vi "15-FindShortestPaths.vi"(5 "Risk Relief":refnum<vi>, 6 "Initial Position in":cluster{"Row":i32, "Col":i32}, 7 "Min Risk Relief":refnum<vi>, 8 "Min Risk Array in":i32[][](array[numeric]), 9 "Visited Array in":bool[][](array[boolean]), 10 "map in":T1(c390), 11 "Risk Array in":u8[][](array[numeric])) -> (0 "Min Risk Array out":i32[][](array[numeric]), 1 "Visited Array out":bool[][](array[boolean]), 2 "map out":T1(c390), 3 "Risk Array out":u8[][](array[numeric]))   [LabVIEW 2019, in "15.lvlib"]
uses:
  15.lvlib
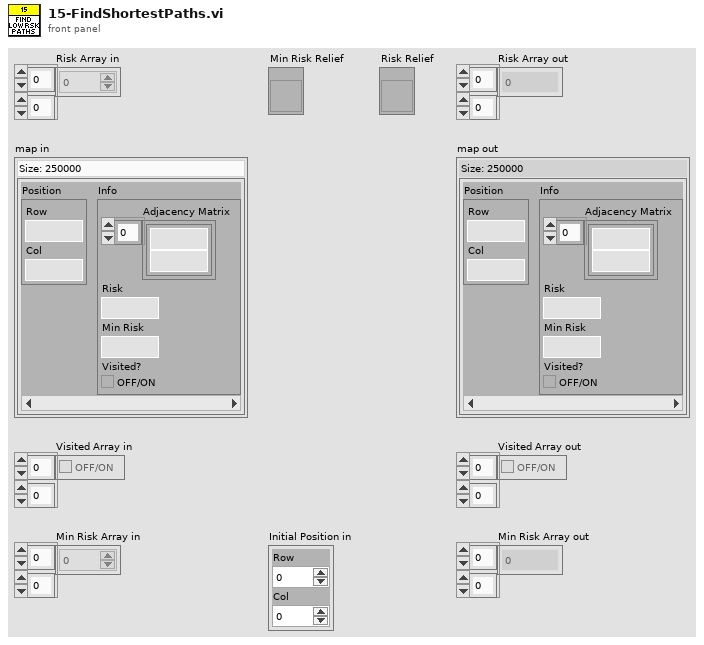
[diagram p1: front panel]
types:
  T1 = map{cluster{"Row":i32, "Col":i32}, cluster{"Adjacency Matrix":cluster{i32, i32}[], "Risk":u8, "Min Risk":i32, "Visited?":bool}}
  T2 = cluster{"Adjacency Matrix":cluster{i32, i32}[], "Risk":u8, "Min Risk":i32, "Visited?":bool}
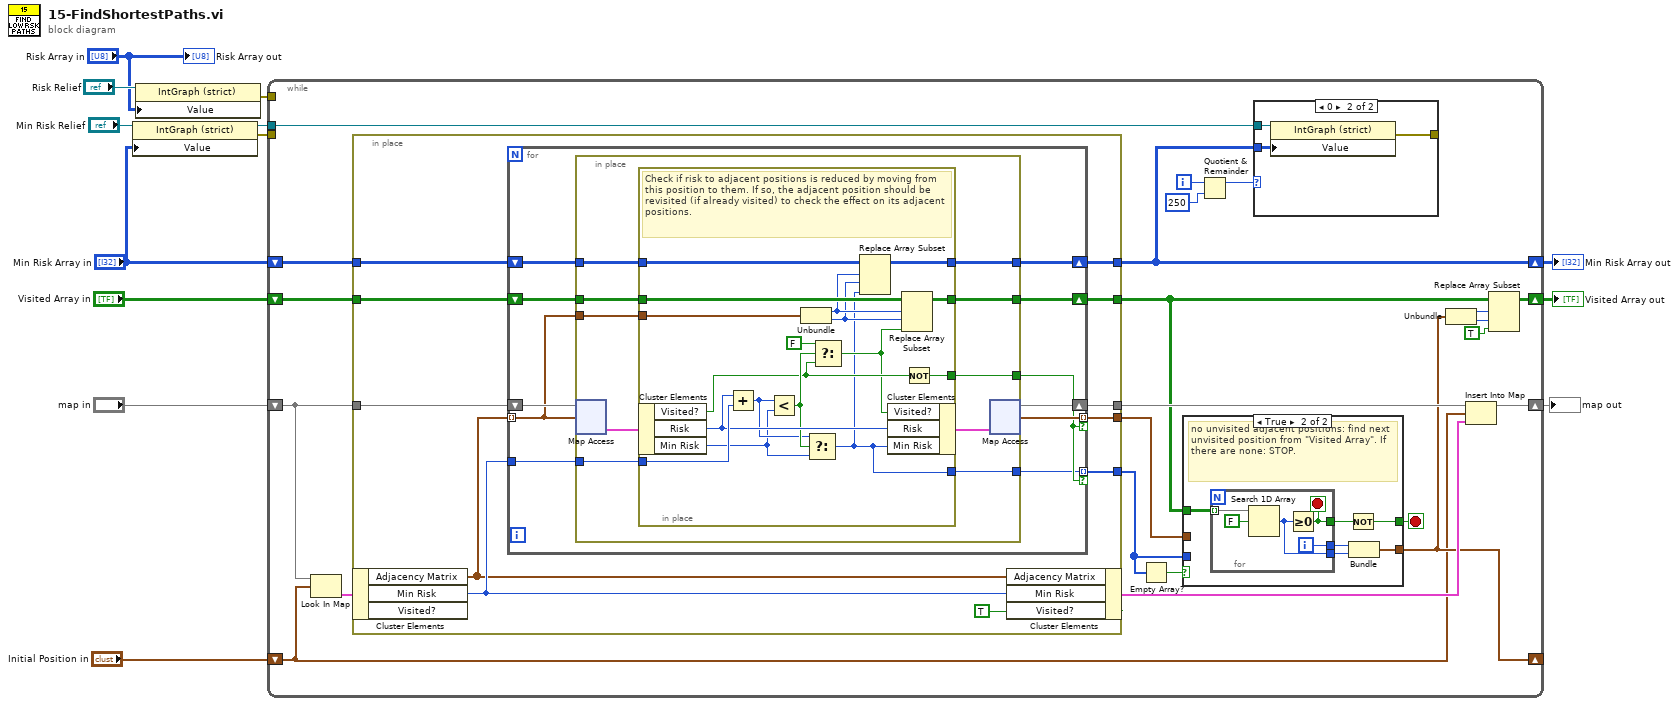
[diagram p0: block diagram]
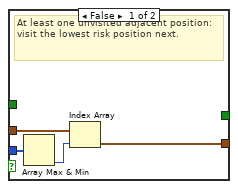
[diagram p3: hidden frame]
diagram:
  n1 = property class="IntGraph (strict)"(reference="Min Risk Relief", "Value"="Min Risk Array in") -> (reference out=w8:refnum<vi>, error out=w2:errorcluster)  [unwired: 1 in]
  n2 = property class="IntGraph (strict)"(reference="Risk Relief", "Value"="Risk Array in") -> (error out=w1:errorcluster)  [unwired: 1 in, 1 out]
  n3 = while {
    shift-right: [w22] -> w11
    shift-left: "map in" -> [w36]
    shift-right: [w27] -> _
    shift-left: "Initial Position in" -> [w24]
    shift-right: [w25] -> w5
    shift-left: "Visited Array in" -> [w21]
    tunnel: w8 -> [w19]
    shift-right: [w17] -> w6
    shift-left: "Min Risk Array in" -> [w18]
    tunnel: w2 -> [_]
    tunnel: w1 -> [_]
    i -> [w16]
    stop <- w23 stop-if-true
    n4 = Look In Map(map=w36, key=w24) -> (value=w35:T2)  [unwired: 1 in, 1 out]
    n5 = in-place {
      in-place-border: w36 -> [w50]
      in-place-border: [w48] -> w34
      in-place-border: [w47] -> w32
      in-place-border: [w46] -> w31
      in-place-border: w21 -> [w45]
      in-place-border: [w44] -> w20
      in-place-border: w18 -> [w41]
      in-place-border: [w40] -> w17
      n6 = in-place-cluster #1(w35) -> ("Adjacency Matrix"=w42:cluster{i32, i32}[], "Min Risk"=w43:i32)  [unwired: 1 out]
      n7 = for {
        shift-right: [w60] -> w48
        shift-left: w50 -> [w61]
        tunnel: w42 -> [w56] mode=indexing
        tunnel: w43 -> [w59]
        tunnel: [w53] -> w46 mode=indexing if=w57
        tunnel: [w58] -> w47 mode=indexing if=w57
        shift-right: [w54] -> w44
        shift-left: w45 -> [w55]
        shift-right: [w51] -> w40
        shift-left: w41 -> [w52]
        n8 = in-place {
          in-place-border: w59 -> [w70]
          in-place-border: [w69] -> w53
          in-place-border: [w68] -> w57
          in-place-border: w56 -> [w66]
          in-place-border: w55 -> [w65]
          in-place-border: [w64] -> w54
          in-place-border: w52 -> [w63]
          in-place-border: [w62] -> w51
          n9 = in-place-map #2(w61, w56) -> (w71:T2)  [unwired: 1 in, 1 out]
          n10 = in-place {
            in-place-border: w70 -> [w88]
            in-place-border: [w72] -> w69
            in-place-border: [w87] -> w68
            in-place-border: w66 -> [w85]
            in-place-border: w65 -> [w83]
            in-place-border: [w82] -> w64
            in-place-border: w63 -> [w76]
            in-place-border: [w75] -> w62
            # "Check if risk to adjacent positions is reduced by moving from this position to them. If so, the adjacent position should be revisited (if already visited) to check the effect on its adjacent positions."
            n11 = in-place-cluster #3(w71) -> ("Visited?"=w78:bool, "Risk"=w86:u8, "Min Risk"=w79:i32)
            n12 = Add(x=w86, y=w88) -> (x+y=w80:i32)
            n13 = Less?(x=w80, y=w79) -> (x < y?=w81:bool)
            n14 = Unbundle(w85) -> (w74:i32, w73:i32)
            n15 = Select(t=w80, s=w81, f=w79) -> (s? t:f=w72:i32)
            n16 = Select(t=FALSE, s=w81, f=w78) -> (s? t:f=w77:bool)
            n17 = Replace Array Subset(array=w76, new element=w72, index (row)=w74, index (col)=w73) -> (w75:i32[][])
            n18 = in-place-cluster #3("Visited?"=w77, "Risk"=w86, "Min Risk"=w72) -> (w67:T2)
            n19 = Replace Array Subset(array=w83, new element=w77, index (row)=w74, index (col)=w73) -> (w82:bool[][])
            n20 = Not(x=w78) -> (.not. x?=w87:bool)
          }
          n21 = in-place-map #2(w67) -> (w60:T1, w58:cluster{"Row":i32, "Col":i32})  [unwired: 1 in, 1 out]
        }
      }
      n22 = in-place-cluster #1("Adjacency Matrix"=w42, "Min Risk"=w43, "Visited?"=TRUE) -> (w33:T2)
    }
    n23 = Empty Array?(array=w31) -> (empty?=w30:bool)
    n24 = case shown="True" w30 {
      tunnel: [w89 w95] -> w27
      tunnel: w32 -> [w91 _]
      tunnel: w31 -> [w90 _]
      tunnel: w20 -> [_ w98]
      tunnel: [_ w93] -> w23
      frame False {
        # "At least one unvisited adjacent position: visit the lowest risk position next."
        n25 = Array Max & Min(array=w90) -> (min index (indices)=w92:i32)  [unwired: 3 out]
        n26 = Index Array(array=w91, index=w92) -> (element=w89:cluster{"Row":i32, "Col":i32})
      }
      frame True {
        # "no unvisited adjacent positions: find next unvisited position from \"Visited Array\". If there are none: STOP."
        n27 = for {
          tunnel: w98 -> [w103] mode=indexing
          tunnel: [w101] -> w97
          tunnel: [w100] -> w96
          tunnel: [w99] -> w94
          i -> [w101]
          stop <- w99 stop-if-true
          n28 = Search 1D Array(1D array=w103, element=FALSE) -> (index of element=w100:i32)  [unwired: 1 in]
          n29 = Greater Or Equal To 0?(x=w100) -> (x >= 0?=w99:bool)
        }
        n30 = Not(x=w94) -> (.not. x?=w93:bool)
        n31 = Bundle(w97, "index of element"=w96) -> (w95:cluster{i32, "index of element":i32})  [unwired: 1 in]
      }
    }
    n32 = Quotient & Remainder(x=w16, y=250) -> (x-y*floor(x/y)=w14:i32)  [unwired: 1 out]
    n33 = case shown="0" w14 {
      tunnel: w19 -> [_ w39]
      tunnel: w17 -> [_ w38]
      tunnel: [_ w37] -> _
      frame Default {
      }
      frame 0 {
        n34 = property class="IntGraph (strict)"(reference=w39, "Value"=w38) -> (error out=w37:errorcluster)  [unwired: 1 in, 1 out]
      }
    }
    n35 = Unbundle(w27) -> ("Row"=w28:i32, "index of element"=w29:i32)
    n36 = Insert Into Map(map in=w34, key=w24, value=w33) -> (map out=w22:T1)  [unwired: 2 out]
    n37 = Replace Array Subset(array=w20, new element=TRUE ("new element/subarray"), index (row)=w28, index (col)=w29) -> (w25:bool[][])
  }
  "map out" <- w11
  "Min Risk Array out" <- w6
  "Visited Array out" <- w5
  "Risk Array out" <- "Risk Array in"
